vi "test bitfile selection.vi"() -> ()   [LabVIEW 2017]
uses:
  <vilib>/addons/InsightCM/Devices/Shared/Common/FpgaBitfileManager/FpgaBitfileManager.lvlib
panel:
  in  "Dynamic Modules":enum16{"2", "3", "6", "8"}(ring)
  in  "9232":bool
  in  "9068":bool
  out "error out":errorcluster
  out "Bitfile":path
  # "9024"
  # "9230"
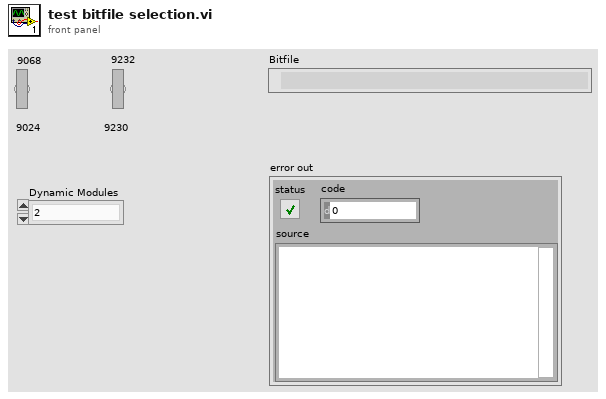
[diagram p1: front panel]
types:
  T1 = typedef "Device.ctl" = cluster{"Id":string, "Name":string, "DeviceType":string, "HardwareName":string, "IpAddress":string, "HardwareInfo":T2, "ApplicationType":string, "ApplicationVersion":string, "EquipmentIds":string[], "ConfigurationVersion":string, "ConfigurationBag":string, "Properties":T2, "DataGroups":T4[]}
  T2 = typedef "KeyValuePairs.ctl" = T3[]
  T3 = typedef "KeyValuePair.ctl" = cluster{"Key":string, "Value":string}
  T4 = typedef "DataGroup.ctl" = cluster{"Name":string, "ChannelIds":string[], "GatingTrigger":T5, "OperatingStates":T7[], "Properties":T2, "EquipmentIds":string[]}
  T5 = typedef "Trigger.ctl" = cluster{"Type":string, "Expression":string, "Conditions":T6[]}
  T6 = typedef "Condition.ctl" = cluster{"Source":string, "Type":string, "Operator":string, "CompareTo":string, "DwellSeconds":dbl}
  T7 = typedef "OperatingState.ctl" = cluster{"Id":string, "Name":string, "StreamMode":bool, "EnterTrigger":T5, "ExitTrigger":T5, "TagCollectionTrigger":T5, "FileCollectionTrigger":T5, "Properties":T2}
  T8 = typedef "cRIODetectHW.lvlib/SystemHW.ctl" = cluster{"controller":T9, "chassis":T9, "modules":T9[]}
  T9 = typedef "cRIODetectHW.lvlib/cRIO Product Info.ctl" = cluster{"vendorName":string, "productName":string, "serialNumber":string}
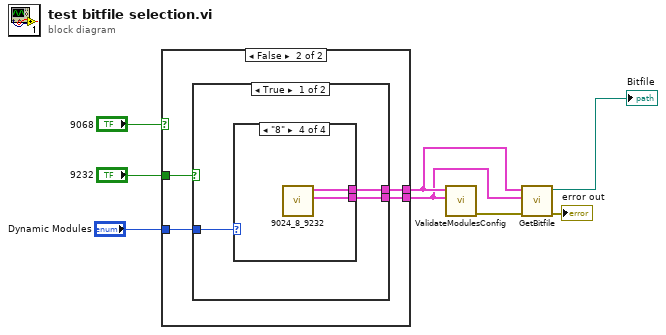
[diagram p0: block diagram]
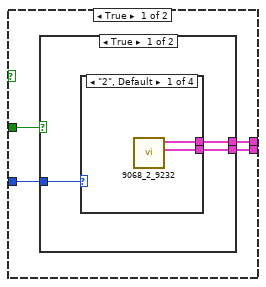
[diagram p2: hidden frame]
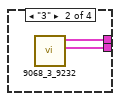
[diagram p3: hidden frame]
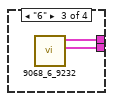
[diagram p4: hidden frame]
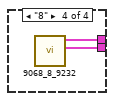
[diagram p5: hidden frame]
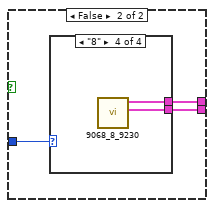
[diagram p6: hidden frame]
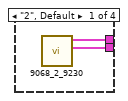
[diagram p7: hidden frame]
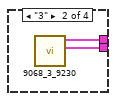
[diagram p8: hidden frame]
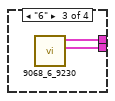
[diagram p9: hidden frame]
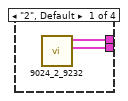
[diagram p10: hidden frame]
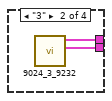
[diagram p11: hidden frame]
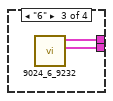
[diagram p12: hidden frame]
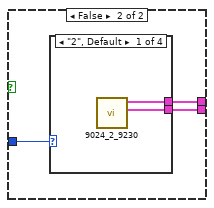
[diagram p13: hidden frame]
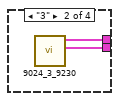
[diagram p14: hidden frame]
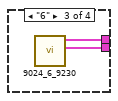
[diagram p15: hidden frame]
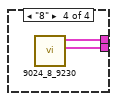
[diagram p16: hidden frame]
diagram:
  n1 = case shown="False" "9068" {
    tunnel: [w12 w38] -> w5
    tunnel: [w11 w37] -> w4
    tunnel: "9232" -> [w10 w36]
    tunnel: "Dynamic Modules" -> [w9 w35]
    frame True {
      n2 = case shown="True" w10 {
        tunnel: [w15 w26] -> w12
        tunnel: [w14 w25] -> w11
        tunnel: w9 -> [w13 w24]
        frame True {
          n3 = case shown="\"2\", Default" w13 {
            tunnel: [w17 w19 w21 w23] -> w15
            tunnel: [w16 w18 w20 w22] -> w14
            frame "2", Default {
              n4 = call <vilib>:"9068_2_9232.vi"() -> ("Device"=w16:T1, "system info"=w17:T8)  [unwired: 10 in]
            }
            frame "3" {
              n5 = call <vilib>:"9068_3_9232.vi"() -> ("Device"=w18:T1, "system info"=w19:T8)  [unwired: 10 in]
            }
            frame "6" {
              n6 = call <vilib>:"9068_6_9232.vi"() -> ("Device"=w20:T1, "system info"=w21:T8)  [unwired: 10 in]
            }
            frame "8" {
              n7 = call <vilib>:"9068_8_9232.vi"() -> ("Device"=w22:T1, "system info"=w23:T8)  [unwired: 10 in]
            }
          }
        }
        frame False {
          n8 = case shown="\"8\"" w24 {
            tunnel: [w28 w30 w32 w34] -> w26
            tunnel: [w27 w29 w31 w33] -> w25
            frame "2", Default {
              n9 = call <vilib>:"9068_2_9230.vi"() -> ("Device"=w27:T1, "system info"=w28:T8)  [unwired: 10 in]
            }
            frame "3" {
              n10 = call <vilib>:"9068_3_9230.vi"() -> ("Device"=w29:T1, "system info"=w30:T8)  [unwired: 10 in]
            }
            frame "6" {
              n11 = call <vilib>:"9068_6_9230.vi"() -> ("Device"=w31:T1, "system info"=w32:T8)  [unwired: 10 in]
            }
            frame "8" {
              n12 = call <vilib>:"9068_8_9230.vi"() -> ("Device"=w33:T1, "system info"=w34:T8)  [unwired: 10 in]
            }
          }
        }
      }
    }
    frame False {
      n13 = case shown="True" w36 {
        tunnel: [w41 w52] -> w38
        tunnel: [w40 w51] -> w37
        tunnel: w35 -> [w39 w50]
        frame True {
          n14 = case shown="\"8\"" w39 {
            tunnel: [w43 w45 w47 w49] -> w41
            tunnel: [w42 w44 w46 w48] -> w40
            frame "2", Default {
              n15 = call <vilib>:"9024_2_9232.vi"() -> ("Device"=w42:T1, "system info"=w43:T8)  [unwired: 10 in]
            }
            frame "3" {
              n16 = call <vilib>:"9024_3_9232.vi"() -> ("Device"=w44:T1, "system info"=w45:T8)  [unwired: 10 in]
            }
            frame "6" {
              n17 = call <vilib>:"9024_6_9232.vi"() -> ("Device"=w46:T1, "system info"=w47:T8)  [unwired: 10 in]
            }
            frame "8" {
              n18 = call <vilib>:"9024_8_9232.vi"() -> ("Device"=w48:T1, "system info"=w49:T8)  [unwired: 10 in]
            }
          }
        }
        frame False {
          n19 = case shown="\"2\", Default" w50 {
            tunnel: [w54 w56 w58 w60] -> w52
            tunnel: [w53 w55 w57 w59] -> w51
            frame "2", Default {
              n20 = call <vilib>:"9024_2_9230.vi"() -> ("Device"=w53:T1, "system info"=w54:T8)  [unwired: 10 in]
            }
            frame "3" {
              n21 = call <vilib>:"9024_3_9230.vi"() -> ("Device"=w55:T1, "system info"=w56:T8)  [unwired: 10 in]
            }
            frame "6" {
              n22 = call <vilib>:"9024_6_9230.vi"() -> ("Device"=w57:T1, "system info"=w58:T8)  [unwired: 10 in]
            }
            frame "8" {
              n23 = call <vilib>:"9024_8_9230.vi"() -> ("Device"=w59:T1, "system info"=w60:T8)  [unwired: 10 in]
            }
          }
        }
      }
    }
  }
  n24 = call <vilib>:"ValidateModulesConfig.vi"("Device"=w4, "system info"=w5) -> ("error out"=w8:errorcluster)  [unwired: 7 in, 2 out]
  n25 = call <vilib>:"GetBitfile.vi"("error in (no error)"=w8, "device"=w4, "system info"=w5) -> ("error out"=→"error out":errorcluster, "Bitfile"=→"Bitfile":path)  [unwired: 7 in]
